vi "Lambda_tau,T,W 2(s').vi"(6 "k":i32, 8 "w":dbl, 9 "T":dbl, 10 "t":dbl, 11 "s'":dbl) -> (3 "L_t,T,W(s')":dbl)   [LabVIEW 2021, in "Phasor.lvlib"]
uses:
  Phasor/Phasor.lvlib
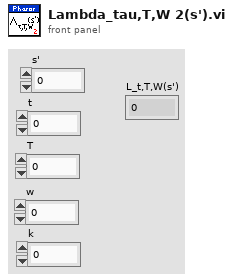
[diagram p1: front panel]
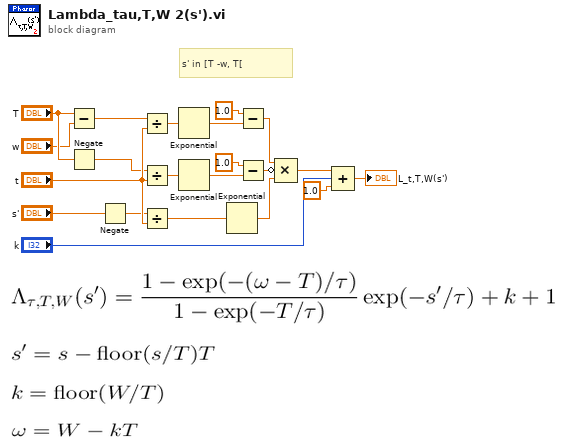
[diagram p0: block diagram]
diagram:
  # "s' in [T -w, T["
  n1 = Subtract(x="T", y="w") -> (x-y=w1:dbl)
  n2 = Negate(x="T") -> (-x=w15:dbl)
  n3 = Negate(x="s'") -> (-x=w10:dbl)
  n4 = Divide(x=w1, y="t") -> (x/y=w18:dbl)
  n5 = Divide(x=w15, y="t") -> (x/y=w14:dbl)
  n6 = Divide(x=w10, y="t") -> (x/y=w9:dbl)
  n7 = Exponential(1:w18) -> (0:w16:dbl)
  n8 = Exponential(1:w14) -> (0:w12:dbl)
  n9 = Exponential(1:w9) -> (0:w8:dbl)
  n10 = Subtract(x=1.0, y=w16) -> (x-y=w7:dbl)
  n11 = Subtract(x=1.0, y=w12) -> (x-y=w6:dbl)
  n12 = Compound Arithmetic op=MULTIPLY(w7, invert w6, w8) -> (w4:dbl)
  n13 = Compound Arithmetic op=ADD(w4, "k", 1.0) -> (→"L_t,T,W(s')":dbl)
